vi "Configure Lamp to Q-Switch Frequency Ratio.vi"(8 "error in (no error)":errorcluster, 10 "ratio":u32, 11 "Lotis in":refnum<class "PL Lotis TII LS.lvclass">) -> (0 "error out":errorcluster, 3 "Lotis out":refnum<class "PL Lotis TII LS.lvclass">)   [LabVIEW 2015, in "PL Lotis TII LS.lvclass"]
doc: "Configures lamp to Q-switch frequency ratio."
uses:
  PL Lotis TII LS.lvclass
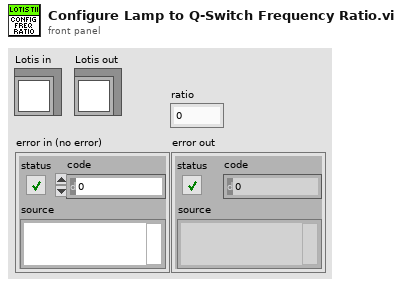
[diagram p1: front panel]
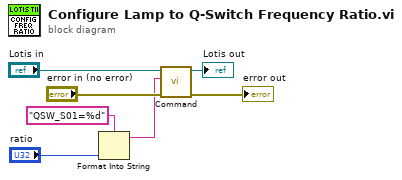
[diagram p0: block diagram]
diagram:
  n1 = Format Into String(format string="QSW_S01=%d" ("command"), "ratio") -> (resulting string=w2:string)  [unwired: 2 in, 1 out]
  n2 = call "Command.vi"("error in (no error)"="error in (no error)", "command"=w2, "Lotis in"="Lotis in") -> ("error out"=→"error out":errorcluster, "Lotis out"=→"Lotis out":refnum<class "PL Lotis TII LS.lvclass">)  [unwired: 6 in, 1 out]
